vi "Main.vi"() -> ()   [LabVIEW 2017]
doc: "Use this template to build a simple state machine design pattern. Each state executes code and determines which state to transition to."
uses:
  controls/State.ctl
  controls/Data.ctl
panel:
  out "Progress":u8(slide) scale=0.0..100.0
  in  "OK Button":bool
  out "Errors":string
  in  "?":T1(tab)
  in  "N6745A":refnum<visa-resource-name>
  in  "KEYSIGHT":refnum<visa-resource-name>
  in  "Set points number by step":bool
  out "Points":dbl caption="Points, N"
  in  "Start":dbl caption="Start, A"
  in  "End":dbl caption="End, A"
  in  "Points Input":dbl caption="Points number"
  out "Step":dbl caption="Step, A"
  in  "Exit":bool
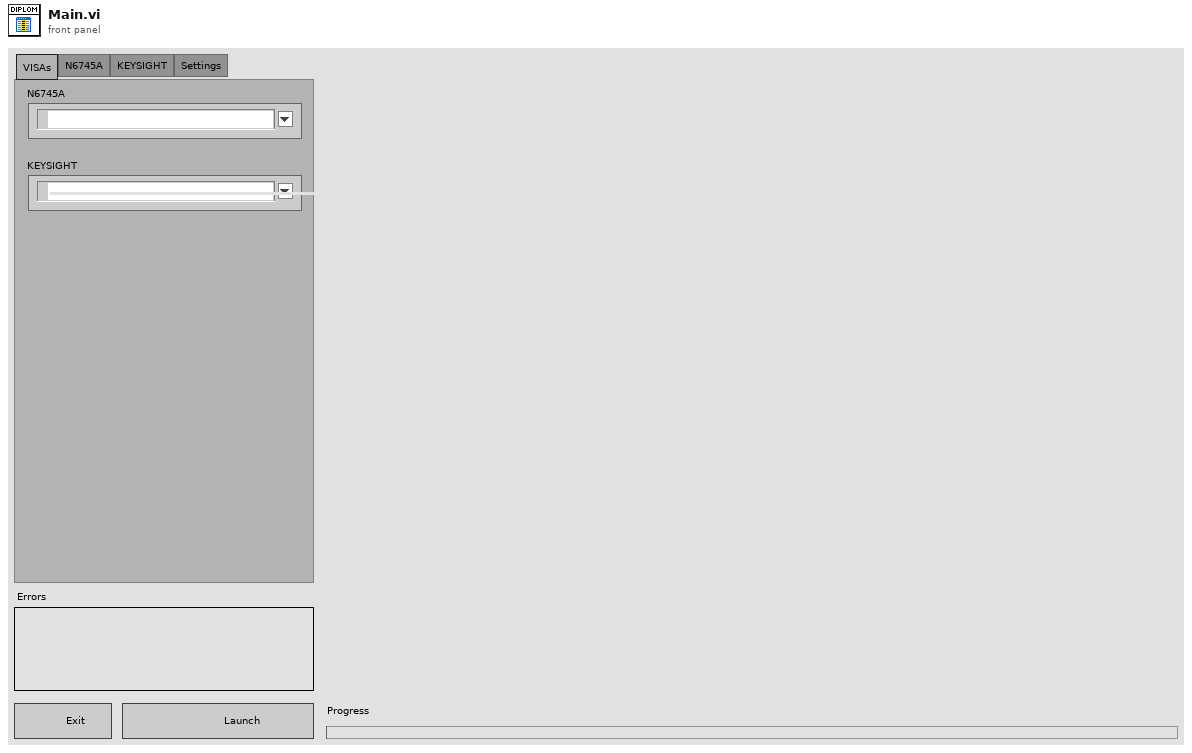
[diagram p1: front panel]
types:
  T1 = enum32{"VISAs", "N6745A", "KEYSIGHT", "Settings"}
  T2 = typedef "Data.ctl" = cluster{"Boolean <Replace Me>":bool, "String <Replace Me>":string, "Numeric <Replace Me>":dbl}
  T3 = typedef "State.ctl" = enum16{"Initialize", "Calculating", "Input", "Init process", "Process", "End process", "Exit"}
  T4 = enum8{"Enabled", "Disabled", "Disabled and Grayed Out"}
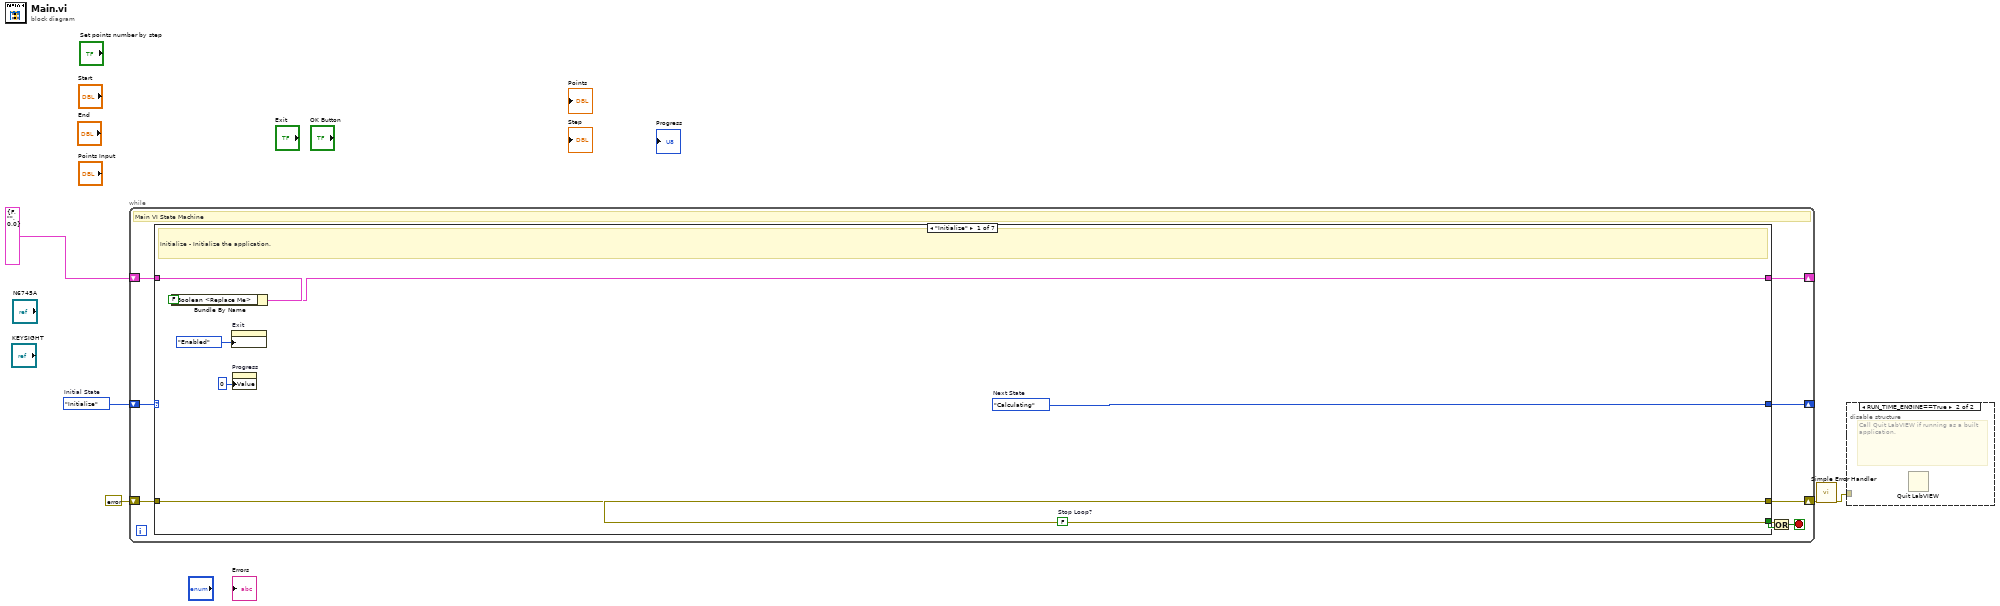
[diagram p0: block diagram]
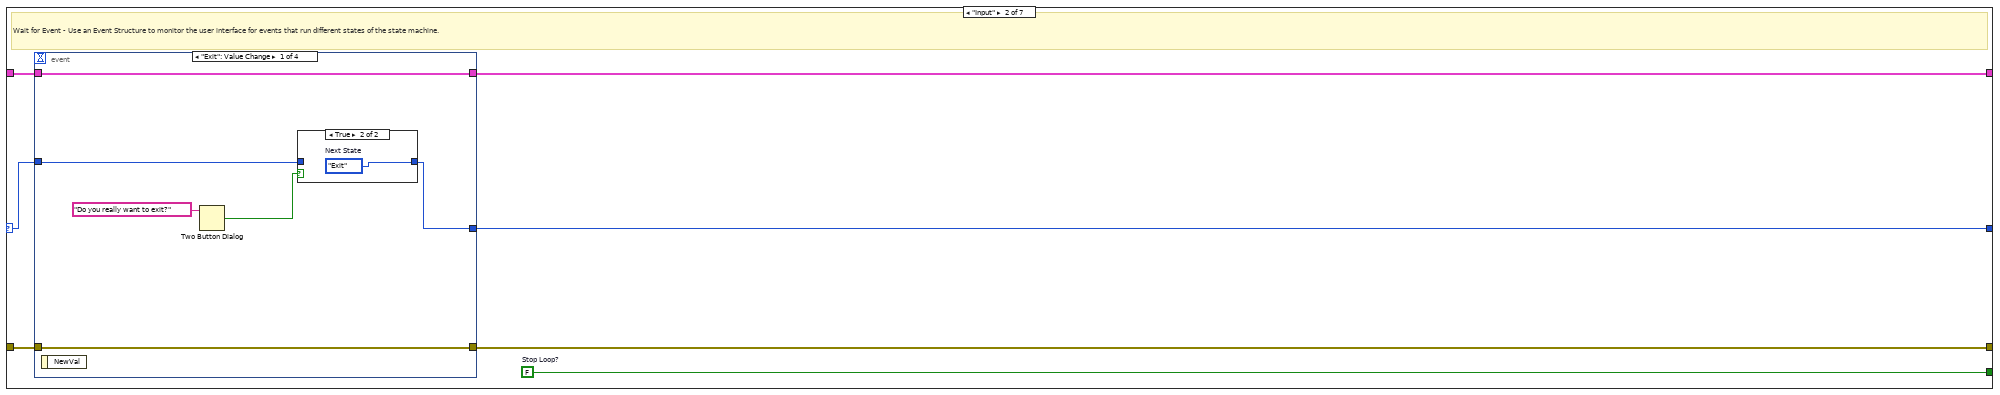
[diagram p3: hidden frame]
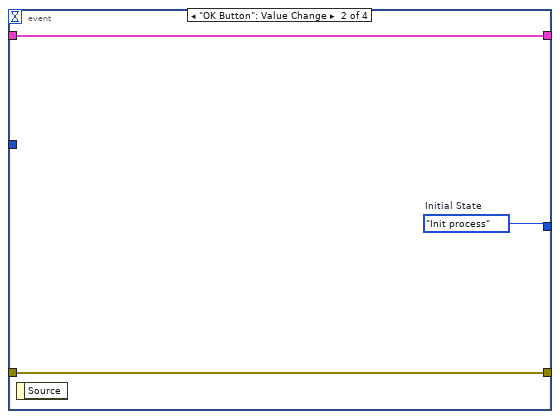
[diagram p5: hidden frame]
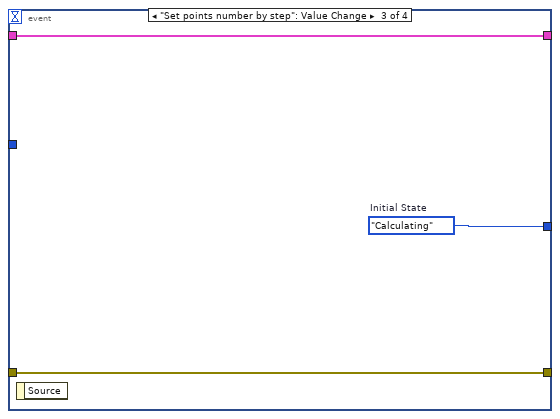
[diagram p6: hidden frame]
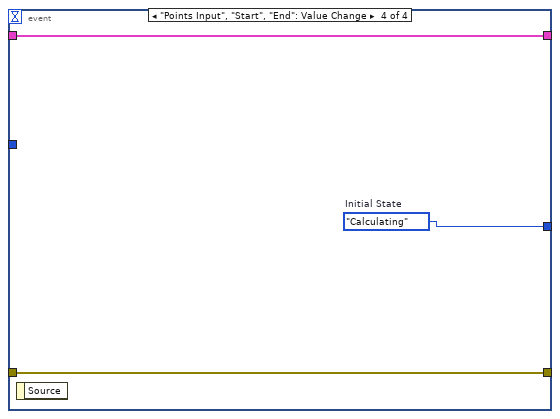
[diagram p7: hidden frame]
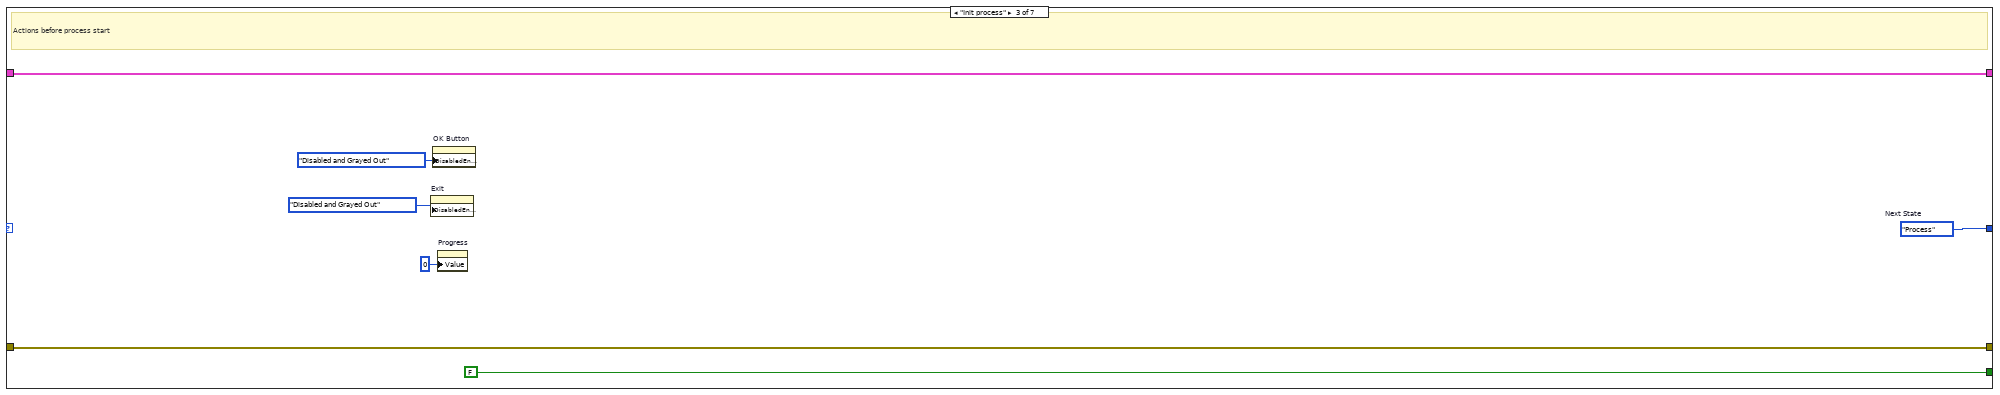
[diagram p8: hidden frame]
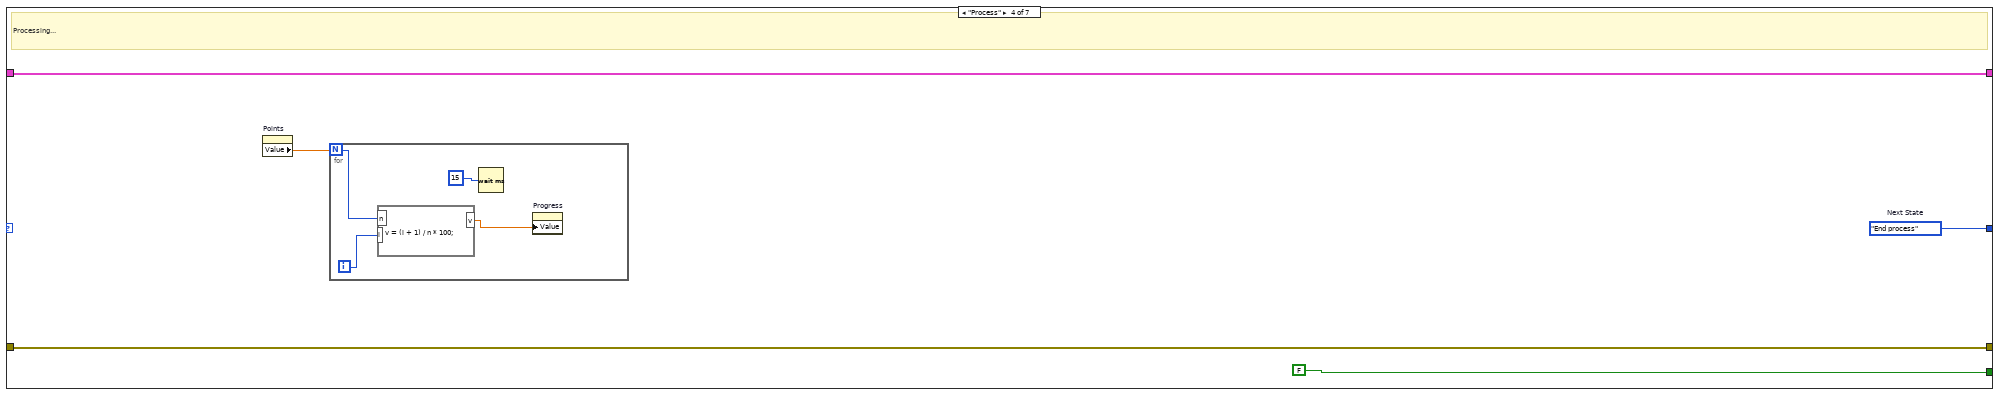
[diagram p9: hidden frame]
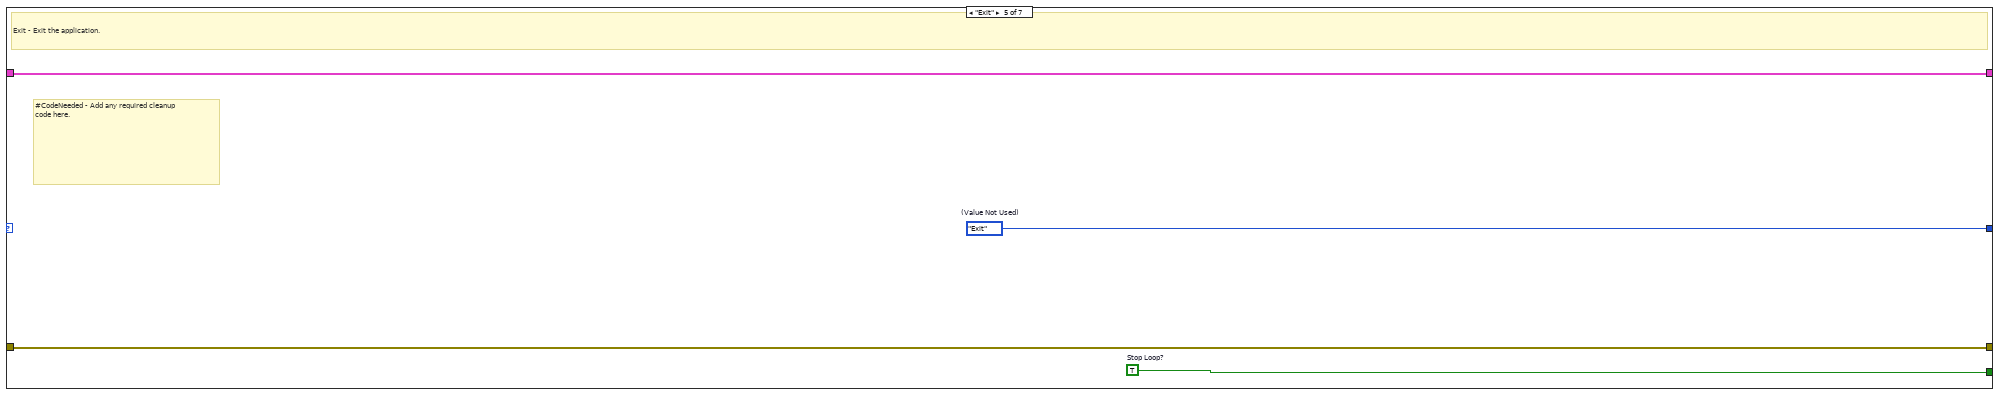
[diagram p10: hidden frame]
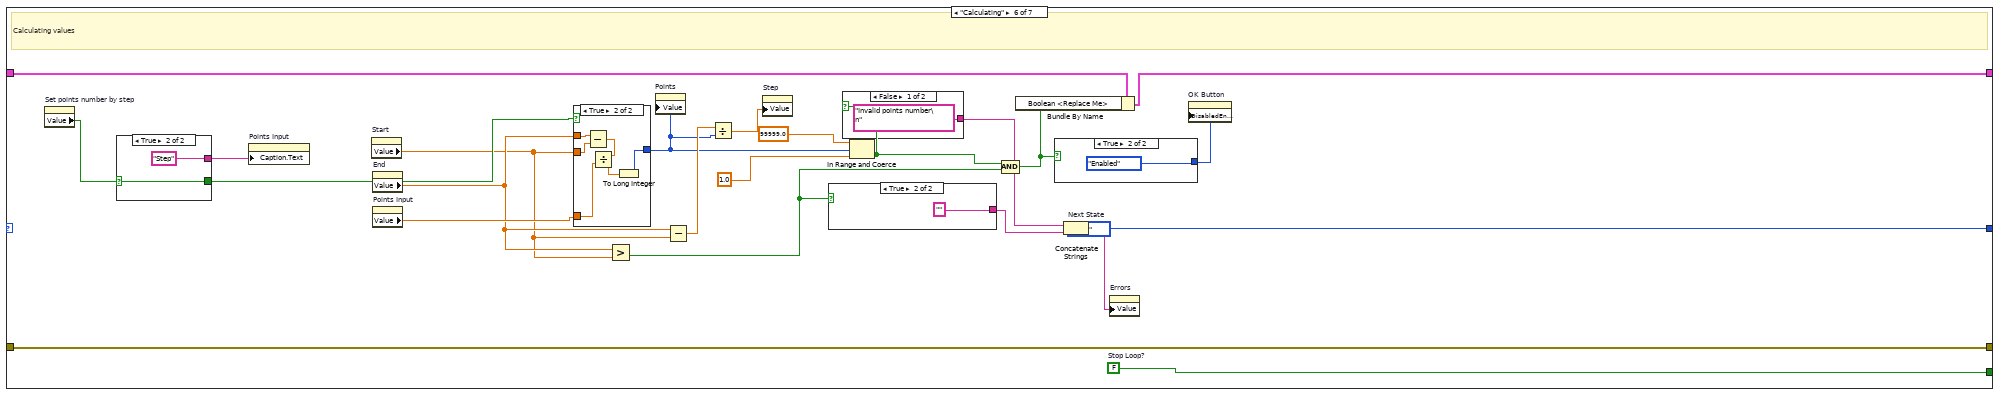
[diagram p11: hidden frame]
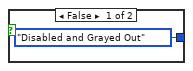
[diagram p12: hidden frame]
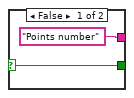
[diagram p13: hidden frame]
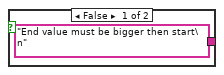
[diagram p14: hidden frame]
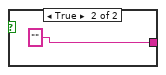
[diagram p15: hidden frame]
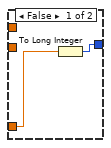
[diagram p16: hidden frame]
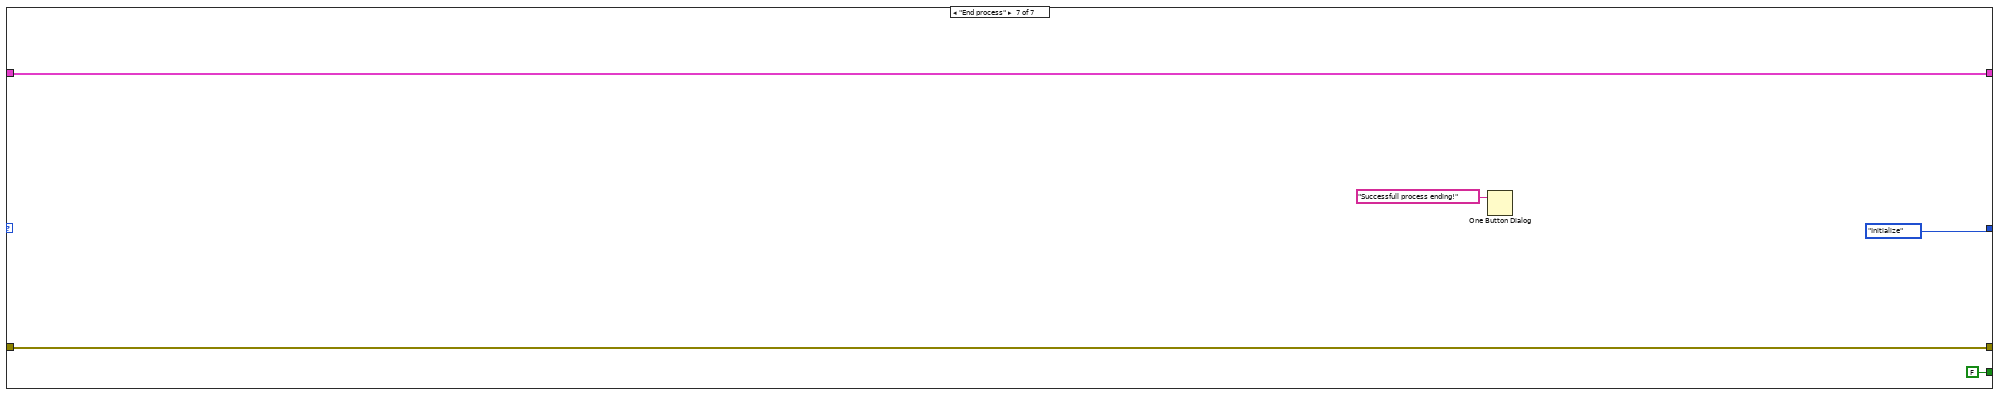
[diagram p17: hidden frame]
diagram:
  w5 = State."Initialize"  # Initial State
  n1 = while {
    shift-right: [w12] -> _
    shift-left: w5 -> [w13]
    shift-right: [w10] -> _
    shift-left: T2 {"Boolean <Replace Me>"=FALSE, "String <Replace Me>"="", "Numeric <Replace Me>"=0.0} ("Data") -> [w11]
    shift-right: [w6] -> w2
    shift-left: errorcluster {"status"=FALSE, "code"=0, "source"=""} ("error constant") -> [w9]
    stop <- w7 stop-if-true
    # "Main VI State Machine"
    n2 = case shown="\"Initialize\"" w13 {
      selector: w13 -> [_ w22 _ _ _ _ _]
      tunnel: [w21 w28 w49 w57 w65 w87 State."Initialize" ("Next State")] -> w12
      tunnel: [w20 w27 FALSE ("Stop Loop?") FALSE ("Stop Loop?") w63 w77 FALSE ("Stop Loop?")] -> w8
      tunnel: w11 -> [w19 w26 w51 w55 w64 w84 w111]
      tunnel: [w18 w25 w51 w55 w64 w83 w111] -> w10
      tunnel: w9 -> [w16 w24 w50 w54 w62 w88 w110]
      tunnel: [w16 w23 w50 w54 w62 w88 w110] -> w6
      frame "Initialize" {
        w20 = FALSE  # Stop Loop?
        w21 = State."Calculating"  # Next State
        # "Initialize - Initialize the application."
        n3 = Bundle By Name(cluster=w19, "Boolean <Replace Me>"=FALSE ("Replace_Me_Boolean")) -> (w18:T2)
        n4 = property on="Exit" class="Bool"("DisabledEnum"=T4."Enabled" ("Disabled")) -> ()  [unwired: 2 in, 2 out]
        n5 = property on="Progress" class="Slide (strict)"("Value"=u8 0 ("Progress")) -> ()  [unwired: 2 in, 2 out]
      }
      frame "Input" {
        w27 = FALSE  # Stop Loop?
        # "Wait for Event - Use an Event Structure to monitor the user interface for events that run different states of the state machine."
        n6 = event shown="[0] \"Exit\": Value Change" {
          selector: _ -> [_ _ _ _]
          dyn-events: _ -> [_ _ _ _]
          timeout: _ -> [_ _ _ _]
          tunnel: [w30 w37 w41 w43] -> w28
          tunnel: w26 -> [w34 w39 w42 w45]
          tunnel: [w34 w39 w42 w45] -> w25
          tunnel: w24 -> [w33 w38 w40 w44]
          tunnel: [w33 w38 w40 w44] -> w23
          tunnel: w22 -> [w31 _ _ _]
          event "Exit": Value Change {
            n7 = event-data() -> ()  [unwired: 1 in, 1 out]
            n8 = Two Button Dialog(message="Do you really want to exit?") -> (T button?=w32:bool)  [unwired: 2 in]
            n9 = case shown="True" w32 {
              tunnel: w31 -> [w35 _]
              tunnel: [w35 w36] -> w30
              frame False {
              }
              frame True {
                w36 = State."Exit"  # Next State
              }
            }
          }
          event "OK Button": Value Change {
            w37 = State."Init process"  # Initial State
            n10 = event-data() -> ()  [unwired: 1 in, 1 out]
          }
          event "Set points number by step": Value Change {
            w41 = State."Calculating"  # Initial State
            n11 = event-data() -> ()  [unwired: 1 in, 1 out]
          }
          event "Points Input", "Start", "End": Value Change {
            w43 = State."Calculating"  # Initial State
            n12 = event-data() -> ()  [unwired: 1 in, 1 out]
          }
        }
      }
      frame "Init process" {
        w49 = State."Process"  # Next State
        # "Actions before process start"
        n13 = property on="Exit" class="Bool"("DisabledEnum"=T4."Disabled and Grayed Out" ("Disabled")) -> ()  [unwired: 2 in, 2 out]
        n14 = property on="OK Button" class="Bool"("DisabledEnum"=T4."Disabled and Grayed Out" ("Disabled")) -> ()  [unwired: 2 in, 2 out]
        n15 = property on="Progress" class="Slide (strict)"("Value"=u8 0 ("Progress")) -> ()  [unwired: 2 in, 2 out]
      }
      frame "Process" {
        w57 = State."End process"  # Next State
        # "Processing..."
        n16 = property on="Points" class="DigNum (strict)"() -> ("Value"=w53:dbl)  [unwired: 2 in, 2 out]
        n17 = for {
          N: w53 -> [w60]
          i -> [w59]
          n18 = formula code="v = (i + 1) / n * 100;"("n"=w60, "i"=w59) -> ("v"=w58:dbl)
          n19 = Wait (ms)(milliseconds to wait=u32 15) -> ()  [unwired: 1 out]
          n20 = property on="Progress" class="Slide (strict)"("Value"=w58) -> ()  [unwired: 2 in, 2 out]
        }
      }
      frame "Exit" {
        w63 = TRUE  # Stop Loop?
        w65 = State."Exit"  # (Value Not Used)
        # "#CodeNeeded - Add any required cleanup code here."
        # "Exit - Exit the application."
      }
      frame "Calculating" {
        w77 = FALSE  # Stop Loop?
        w87 = State."Input"  # Next State
        # "Calculating values"
        n21 = property on="Set points number by step" class="Bool (strict)"() -> ("Value"=w76:bool)  [unwired: 2 in, 2 out]
        n22 = case shown="True" w76 {
          selector: w76 -> [w91 w93]
          tunnel: ["Points number" "Step"] -> w74
          tunnel: [w91 w93] -> w75
          frame False {
          }
          frame True {
          }
        }
        n23 = property on="Points Input" class="DigNum (strict)"("Caption.Text"=w74) -> ()  [unwired: 2 in, 2 out]
        n24 = property on="Start" class="DigNum (strict)"() -> ("Value"=w72:dbl)  [unwired: 2 in, 2 out]
        n25 = property on="End" class="DigNum (strict)"() -> ("Value"=w73:dbl)  [unwired: 2 in, 2 out]
        n26 = property on="Points Input" class="DigNum (strict)"() -> ("Value"=w86:dbl)  [unwired: 2 in, 2 out]
        n27 = case shown="True" w75 {
          tunnel: w73 -> [_ w106]
          tunnel: w72 -> [_ w105]
          tunnel: w86 -> [w100 w103]
          tunnel: [w99 w101] -> w70
          frame False {
            n28 = To Long Integer(number=w100) -> (32bit integer=w99:i32)
          }
          frame True {
            n29 = Subtract(x=w106, y=w105) -> (x-y=w104:dbl)
            n30 = Divide(x=w104, y=w103) -> (x/y=w102:dbl)
            n31 = To Long Integer(number=w102) -> (32bit integer=w101:i32)
          }
        }
        n32 = Greater?(x=w73, y=w72) -> (0:w79:bool)
        n33 = property on="Points" class="DigNum (strict)"("Value"=w70) -> ()  [unwired: 2 in, 2 out]
        n34 = Subtract(x=w73, y=w72) -> (x-y=w71:dbl)
        n35 = Divide(x=w71, y=w70) -> (x/y=w69:dbl)
        n36 = property on="Step" class="DigNum (strict)"("Value"=w69) -> ()  [unwired: 2 in, 2 out]
        n37 = case shown="True" w79 {
          tunnel: ["End value must be bigger then start\n" ""] -> w78
          frame False {
          }
          frame True {
          }
        }
        n38 = In Range and Coerce(upper limit=99999.0, x=w70, lower limit=1.0) -> (In Range?=w82:bool)  [unwired: 1 out]
        n39 = case shown="False" w82 {
          tunnel: ["Invalid points number\n" ""] -> w81
          frame False {
          }
          frame True {
          }
        }
        n40 = Compound Arithmetic op=AND(w82, w79) -> (w68:bool)
        n41 = Bundle By Name(cluster=w84, "Boolean <Replace Me>"=w68) -> (w83:T2)
        n42 = case shown="True" w68 {
          tunnel: [T4."Disabled and Grayed Out" ("Disabled") T4."Enabled" ("Disabled")] -> w67
          frame False {
          }
          frame True {
          }
        }
        n43 = Concatenate Strings(w81, w78) -> (w80:string)
        n44 = property on="Errors" class="Str"("Value"=w80) -> ()  [unwired: 2 in, 2 out]
        n45 = property on="OK Button" class="Bool"("DisabledEnum"=w67) -> ()  [unwired: 2 in, 2 out]
      }
      frame "End process" {
        n46 = One Button Dialog(message="Successfull process ending!") -> ()  [unwired: 1 in, 1 out]
      }
    }
    n47 = Or(x=w6, y=w8) -> (x .or. y?=w7:bool)
  }
  n48 = call <vilib>:"Simple Error Handler.vi"("error in (no error)"=w2) -> ("error out"=w1:errorcluster)  [unwired: 4 in, 4 out]
  n49 = disable-structure shown="RUN_TIME_ENGINE==True" {
    disable-tunnel: w1 -> [_ _]
    frame condition #0 (active) {
    }
    frame condition #1 {
      # "Call Quit LabVIEW if running as a built application."
      n50 = Quit LabVIEW() -> ()  [unwired: 1 in]
    }
  }
